vi "DHE_DRV_stop_exposure.vi"(0 "fd":i32, 11 "error in (no error)":errorcluster) -> (4 "fd out":i32, 6 "read val":i32, 15 "error out":errorcluster)   [LabVIEW 2016]
doc: "This VI closes the I/O interface with the instrument."
uses:
  c/lib/libarcDHE.so
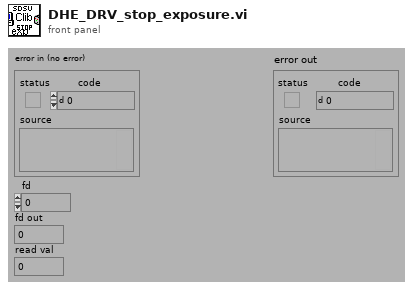
[diagram p1: front panel]
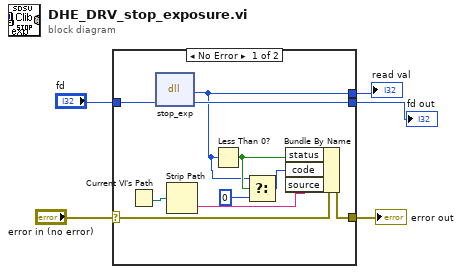
[diagram p0: block diagram]
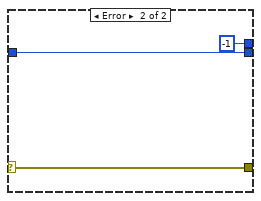
[diagram p2: hidden frame]
diagram:
  n1 = case shown="No Error" "error in (no error)" {
    selector: "error in (no error)" -> [w12 w17]
    tunnel: [w13 w17] -> w5
    tunnel: "fd" -> [w11 w18]
    tunnel: [w10 w18] -> w2
    tunnel: [w8 -1] -> w1
    frame No Error {
      n2 = Current VI's Path() -> (path=w15:path)
      n3 = dll-call lib="home/simager/panview/PAN/Modules/SDSU/private/c/lib/libarcDHE.so" fn="stop_exp" label="stop_exposure"("fd"=w11) -> (w8:i32, "fd"=w10:i32)  [unwired: 3 in, 2 out]
      n4 = Strip Path(path=w15) -> (name=w14:string)  [unwired: 1 out]
      n5 = Less Than 0?(x=w8) -> (x < 0?=w9:bool)
      n6 = Select(t=w8, s=w9, f=0) -> (s? t:f=w6:i32)
      n7 = Bundle By Name(cluster=w12, "status"=w9, "code"=w6, "source"=w14) -> (w13:errorcluster)
    }
    frame Error {
    }
  }
  "error out" <- w5
  "fd out" <- w2
  "read val" <- w1
